vi "Get Sampling Point.vi"(8 "error in (no error)":errorcluster, 10 "position":u8, 11 "Distance IR Bricklet in":refnum<class "Distance IR Bricklet.lvclass">) -> (0 "error out":errorcluster, 2 "distance":u16, 3 "Distance IR Bricklet out":refnum<class "Distance IR Bricklet.lvclass">)   [LabVIEW 2011, in "Tinkerforge.lvlib" / "Distance IR Bricklet.lvclass"]
doc: "This VI returns the distance to a sampling point position as set by \"Set Sampling Point.vi\"."
uses:
  Distance IR Bricklet.lvclass
  Device/Device.lvclass
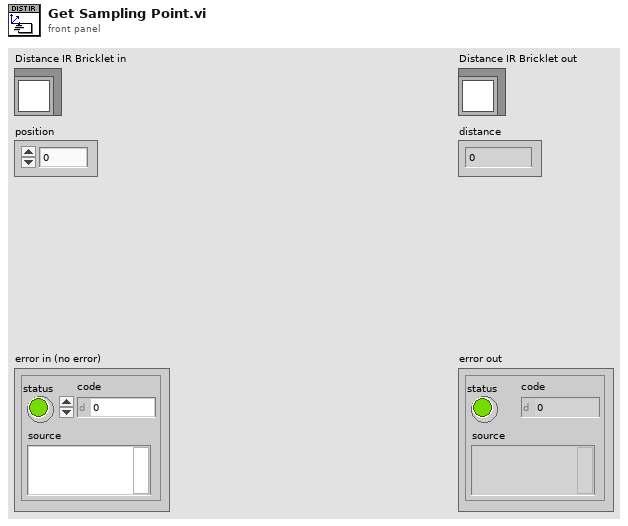
[diagram p1: front panel]
types:
  T1 = typedef "Tinkerforge.lvlib/IP Connection.lvclass/Answer.ctl" = cluster{"Request GUID":string, "Request Type":T2, "Sucessful":bool, "Data":variant, "Error":errorcluster}
  T2 = typedef "Tinkerforge.lvlib/IP Connection.lvclass/Request Type.ctl" = enum8{"Invalid", "Write"}
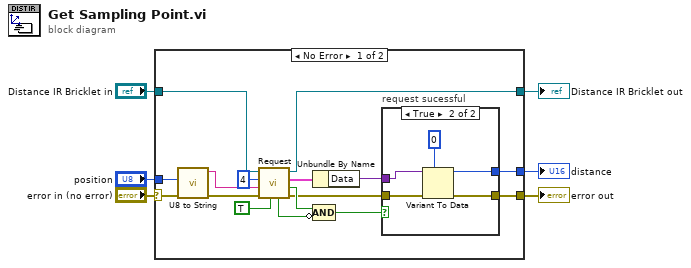
[diagram p0: block diagram]
diagram:
  n1 = case shown="No Error" "error in (no error)" {
    selector: "error in (no error)" -> [w11 w30]
    tunnel: [w12 w30] -> w5
    tunnel: [w21 w29] -> w3
    tunnel: "Distance IR Bricklet in" -> [w22 w29]
    tunnel: [w7 _] -> w2
    tunnel: "position" -> [w8 _]
    frame No Error {
      n2 = call "U8 to String.vi"("Error In"=w11, "U8"=w8) -> ("Error Out"=w10:errorcluster, "String out"=w9:string)  [unwired: 8 in]
      n3 = call "Request.vi"("Response"=TRUE, "error in (no error)"=w10, "Data"=w9, "Function ID"=u8 4, "Device in"=w22) -> ("error out"=w15:errorcluster, "Sucessful"=w17:bool, "Answer"=w14:T1, "Device out"=w21:refnum<class "Distance IR Bricklet.lvclass">, "timed out"=w18:bool)  [unwired: 2 in]
      n4 = Unbundle By Name(w14) -> ("Data"=w13:variant)
      n5 = Compound Arithmetic op=AND(w17, invert w18) -> (w16:bool)
      n6 = case "request sucessful" shown="True" w16 {
        tunnel: w15 -> [w23 w28]
        tunnel: w13 -> [_ w26]
        tunnel: [_ w25] -> w7
        tunnel: [w23 w24] -> w12
        frame False {
        }
        frame True {
          n7 = Variant To Data(error in=w28, type=u16 0, Variant=w26) -> (data=w25:u16, error out=w24:errorcluster)
        }
      }
    }
    frame Error {
    }
  }
  "error out" <- w5
  "Distance IR Bricklet out" <- w3
  "distance" <- w2
